vi "New Heading 2 Object.vi"(8 "error in (no error)":errorcluster) -> (0 "error out":errorcluster, 3 "Heading 2 out":refnum<class "Heading 2.lvclass">)   [LabVIEW 2017, in "Styles.lvlib" / "Heading 2.lvclass"]
uses:
  Heading 2.lvclass
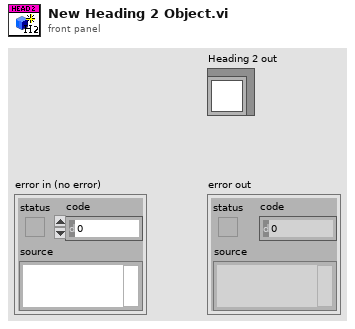
[diagram p1: front panel]
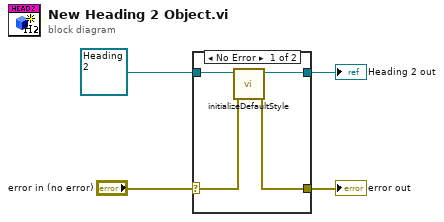
[diagram p0: block diagram]
diagram:
  n1 = case shown="No Error" "error in (no error)" {
    selector: "error in (no error)" -> [w7 w10]
    tunnel: refnum<class "Heading 2.lvclass"> refnum ("Heading 2 in") -> [w8 w9]
    tunnel: [w6 w10] -> w1
    tunnel: [w5 w9] -> w3
    frame No Error {
      n2 = call-dynamic "initializeDefaultStyle.vi"("error in (no error)"=w7, "Heading 2 in"=w8) -> ("error out"=w6:errorcluster, "Heading 2 out"=w5:refnum<class "Heading 2.lvclass">)  [unwired: 8 in]
    }
    frame Error {
    }
  }
  "error out" <- w1
  "Heading 2 out" <- w3
